vi "visa_test.vi"   [LabVIEW 2019]
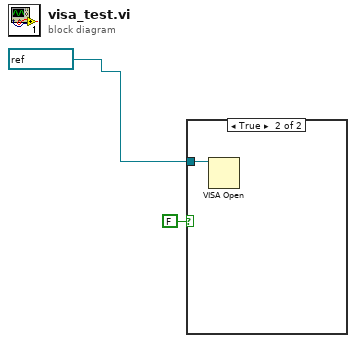
[diagram p0: block diagram]
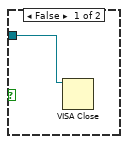
[diagram p2: hidden frame]
diagram:
  n1 = case shown="True" FALSE {
    tunnel: refnum<visa-resource-name> "COM4" ("VISA resource name") -> [w3 w4]
    frame False {
      n2 = VISA Close(VISA resource name=w3) -> ()  [unwired: 1 in, 1 out]
    }
    frame True {
      n3 = VISA Open(VISA resource name=w4) -> ()  [unwired: 4 in, 2 out]
    }
  }
